vi "parse_arduino_data_message (sub-vi).vi"(8 "error in":errorcluster, 9 "format string (%f)":string, 10 "data label":string, 11 "input string":string) -> (0 "error out":errorcluster, 2 "array out":dbl[](array[numeric]), 3 "match length":i32)   [LabVIEW 2021]
uses:
  <vilib>/regexp/Match Regular Expression.xnode
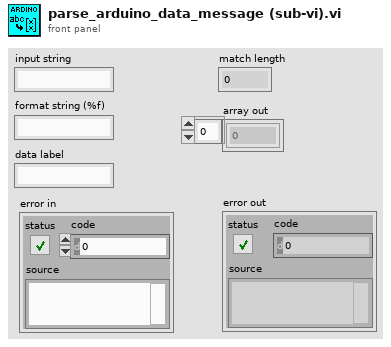
[diagram p1: front panel]
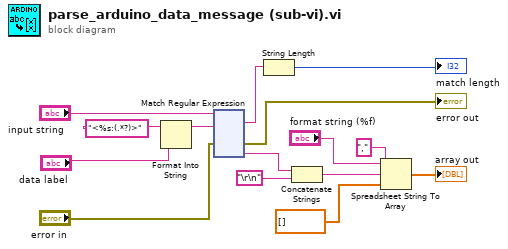
[diagram p0: block diagram]
diagram:
  n1 = Format Into String(format string="<%s:(.*?)>", "data label") -> (resulting string=w6:string)  [unwired: 2 in, 1 out]
  n2 = xnode "Match Regular Expression"("input string"="input string", "regular expression"=w6, "error in"="error in") -> ("whole match"=w10:string, "error out"=→"error out":errorcluster, "submatch 1"=w5:string)  [unwired: 3 in, 3 out]
  n3 = String Length(string=w10) -> (length=→"match length":i32)
  n4 = Concatenate Strings(w5, "\r\n") -> (w3:string)
  n5 = Spreadsheet String To Array(delimiter (Tab)=",", format string="format string (%f)", spreadsheet string=w3, array type (2D Dbl)=dbl[] []) -> (array=→"array out":dbl[])
